vi "Automatic Teller Machine (ATM).vi"() -> ()   [LabVIEW 2020]
doc: "This is my ATM machine"
uses:
  Controls/Ctrl_states.ctl
  Controls/Ctrl_local.ctl
  Controls/Ctrl_UI_Ref.ctl
  <vilib>/Utility/file.llb/Read Delimited Spreadsheet (string).vi
  <vilib>/Utility/file.llb/Write Delimited Spreadsheet (string).vi
panel:
  in  "Enter":bool
  in  "User Input":string
  in  "Right Buttons":T1
  out "Right Menu":T2
  in  "Left Buttons":T1
  out "Left Menu":T2
  in  "Card Simulator":bool
  out "ATM Messages":string
  out "error out":errorcluster caption="sortie d'erreur"
  in  "error in":errorcluster caption="entrée d'erreur"
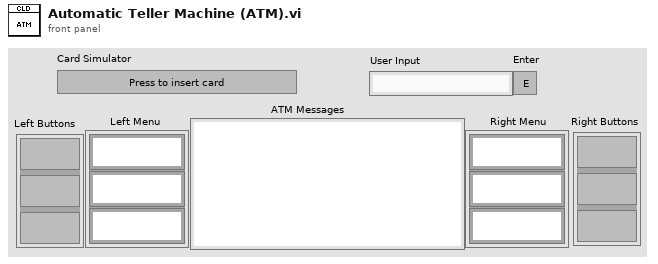
[diagram p1: front panel]
types:
  T1 = cluster{"Func Button":bool, "Func Button 2":bool, "Func Button 3":bool}
  T2 = cluster{"RFS String":string, "RFS String 2":string, "RFS String 3":string}
  T3 = typedef "Ctrl_states.ctl" = enum16{"Account exist", "Account not exist", "Balance Inquiry", "Card inserted", "Display", "Deposit", "Error", "Enter", "Fast Cash", "Read FIle", "Idle", "Init", "Return Card and Terminate", "Save file", "Stop", "Start", "Terminate", "Withdraw"}
  T4 = enum8{"Enabled", "Disabled", "Disabled and Grayed Out"}
  T5 = typedef "Ctrl_local.ctl" = cluster{"State":T3, "Ref":T6, "ATM message":string, "Data":string[][], "User_Input":string, "User_idx":i32, "Terminate ?":bool, "Left Menu":cluster{"RFS String":string, "RFS String 2":string, "RFS String 3":string}, "Right Menu":cluster{"RFS String":string, "RFS String 2":string, "RFS String 3":string}, "Context":T3, "File path":path, "error in":errorcluster}
  T6 = typedef "Ctrl_UI_Ref.ctl" = cluster{"User Input":refnum<vi>, "Enter":refnum<vi>, "Right Buttons":refnum<vi>, "Right Menu":refnum<vi>, "Left Buttons":refnum<vi>, "Left Menu":refnum<vi>, "Card Simulator":refnum<vi>}
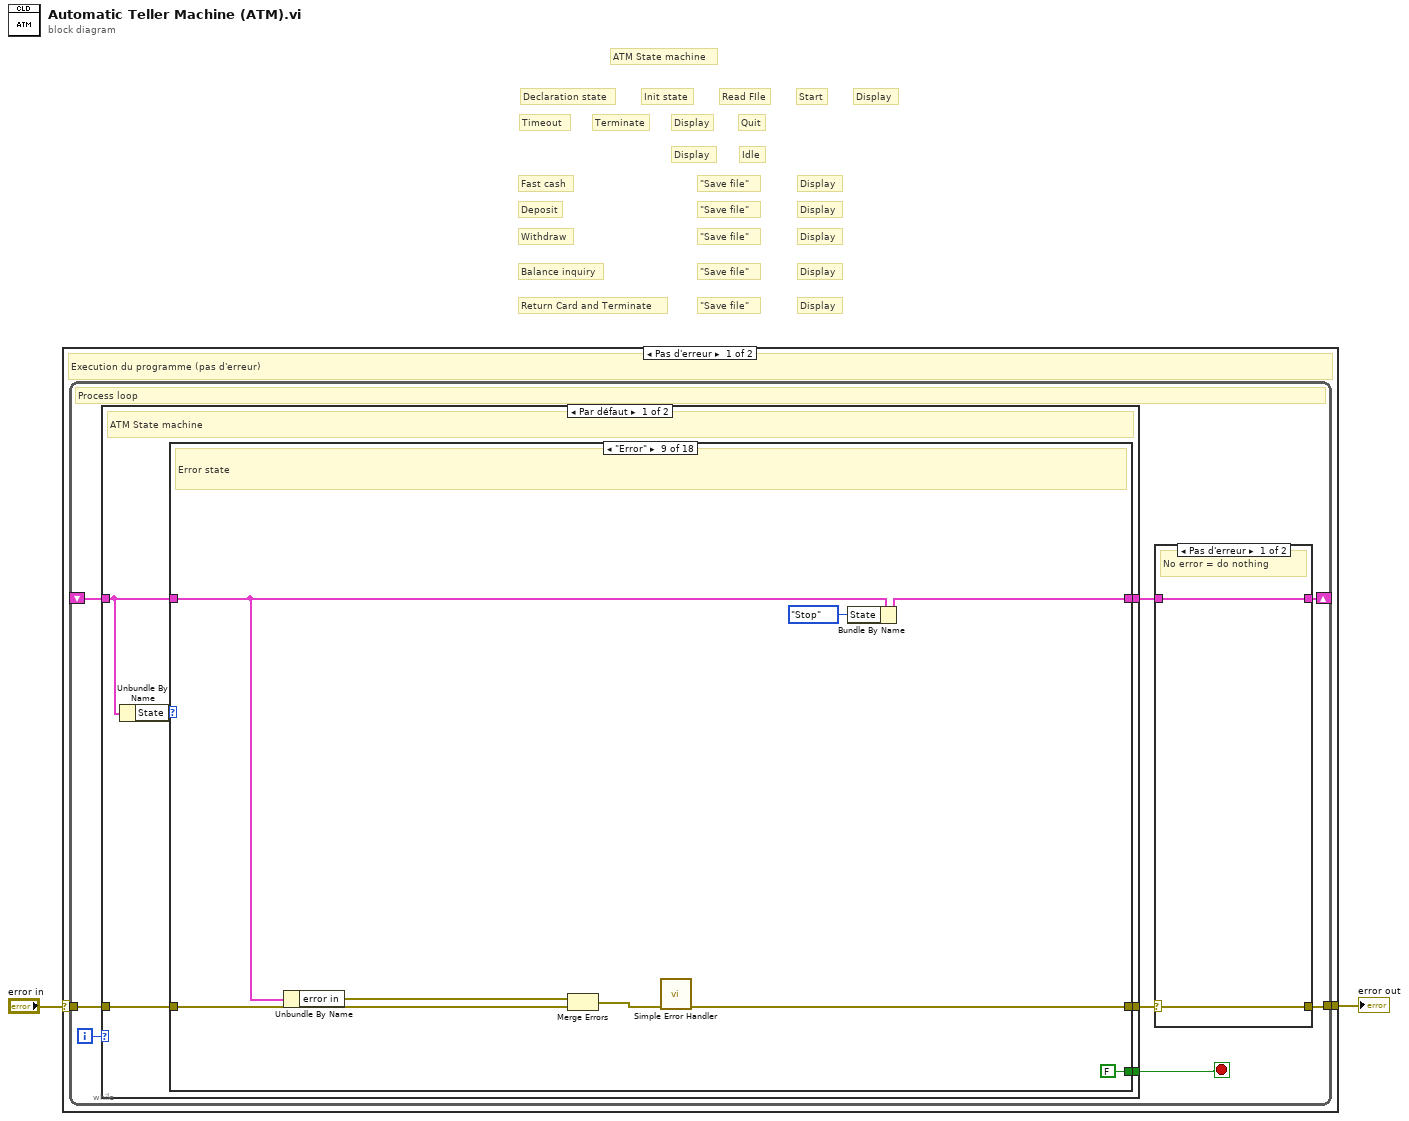
[diagram p0: block diagram]
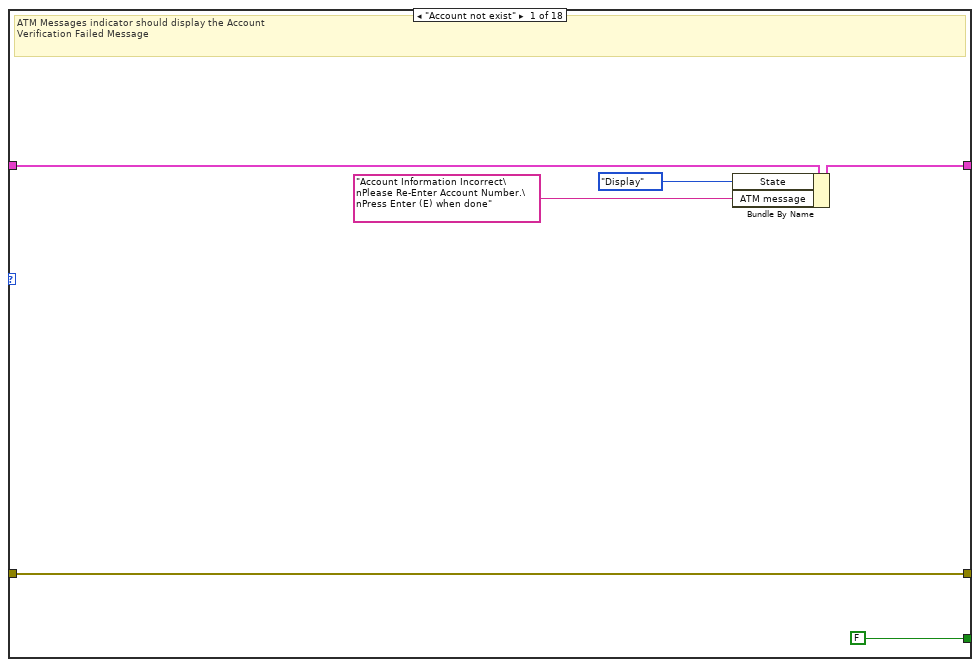
[diagram p2: hidden frame]
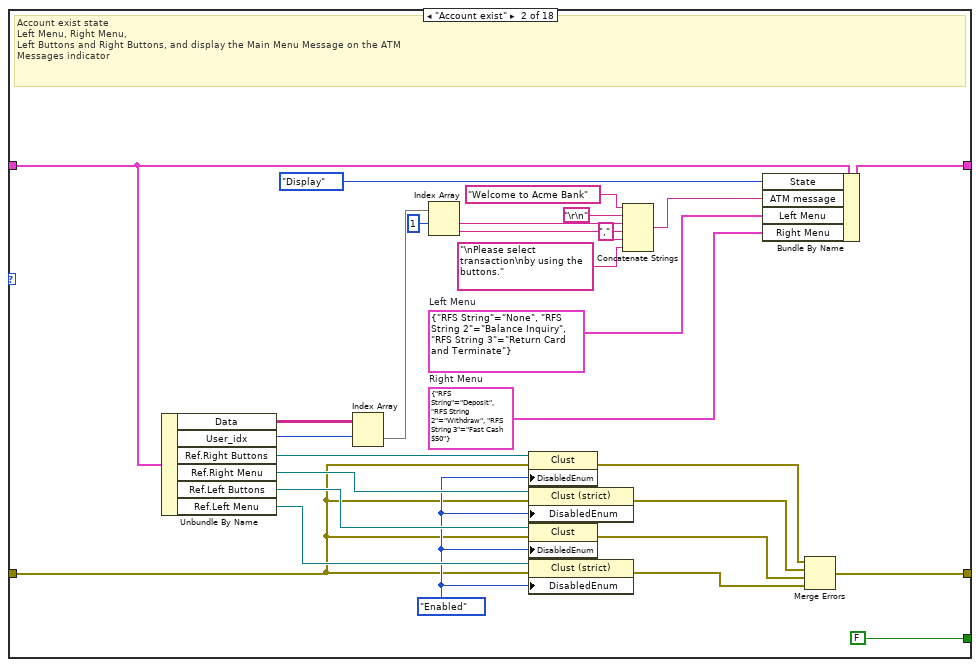
[diagram p3: hidden frame]
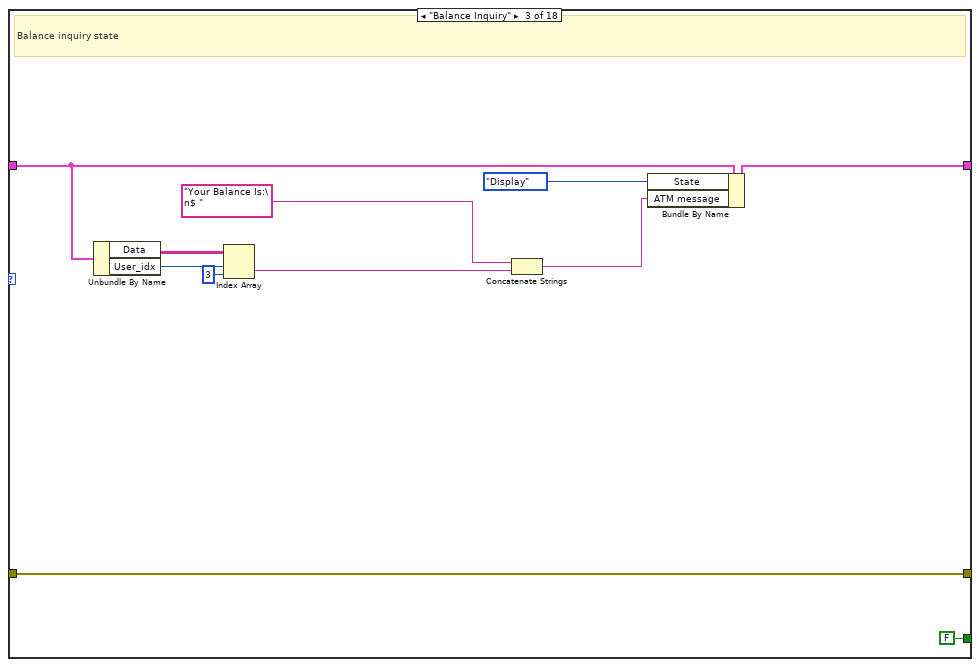
[diagram p4: hidden frame]
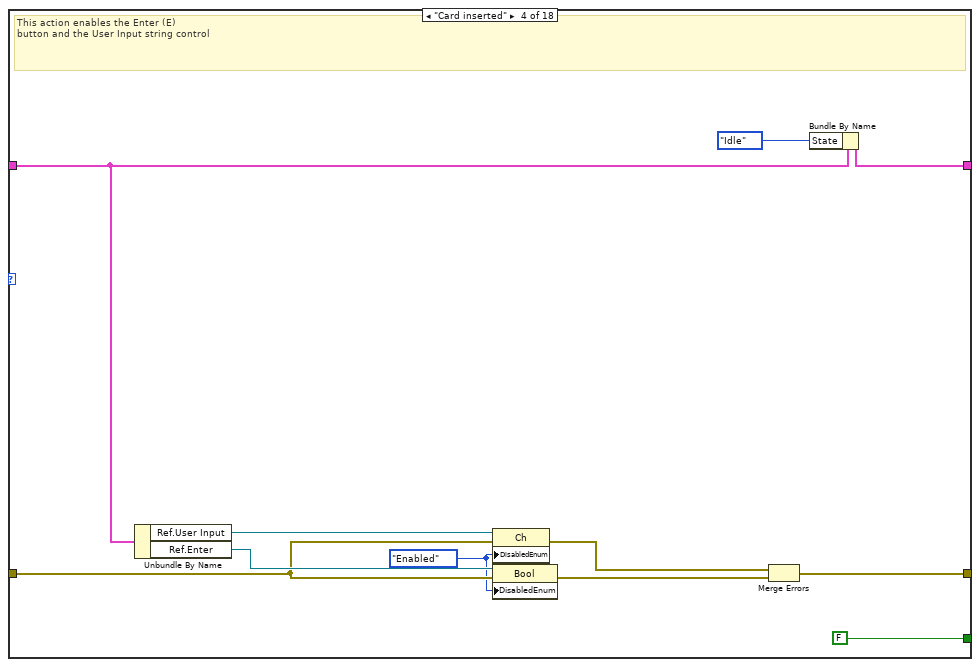
[diagram p5: hidden frame]
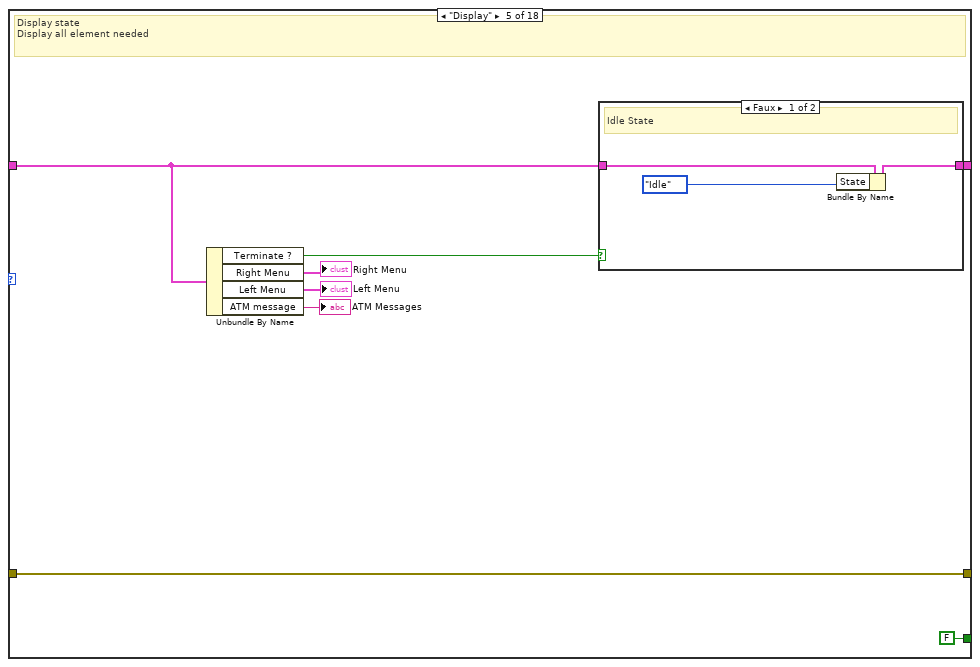
[diagram p6: hidden frame]
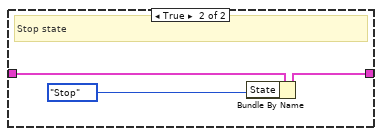
[diagram p7: hidden frame]
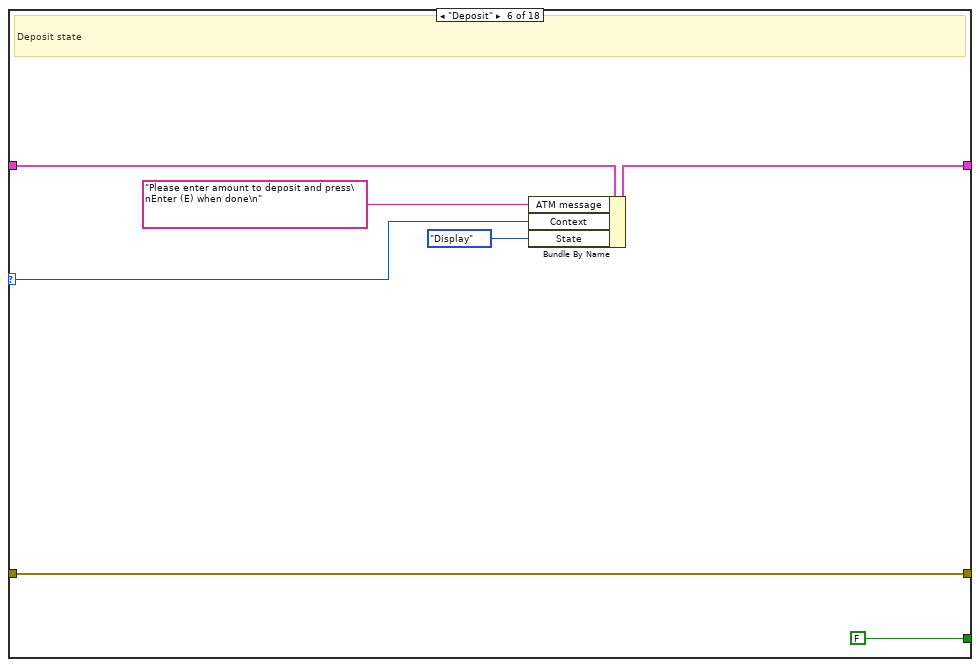
[diagram p8: hidden frame]
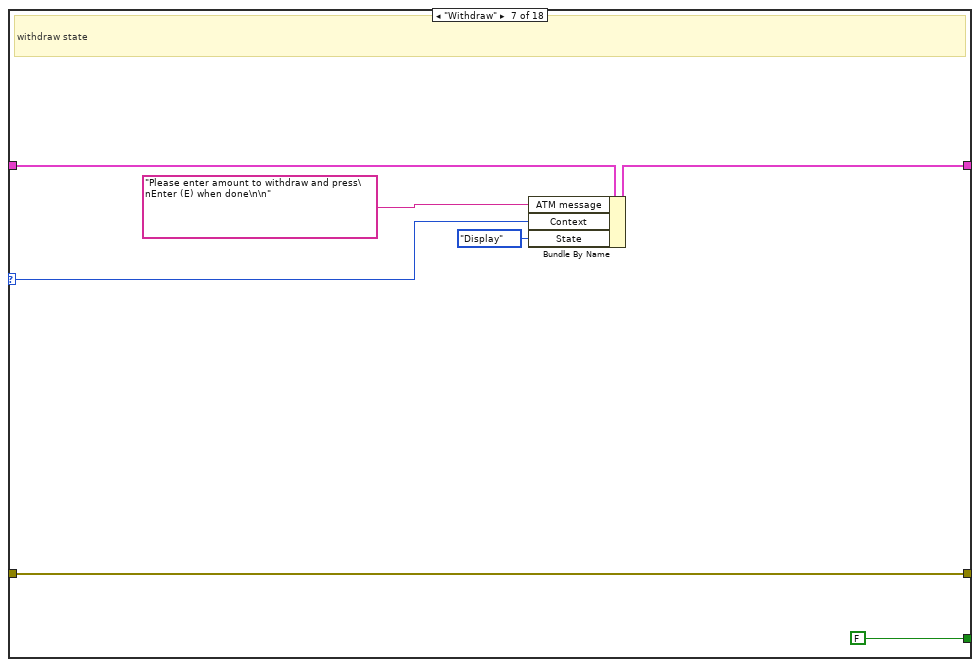
[diagram p9: hidden frame]
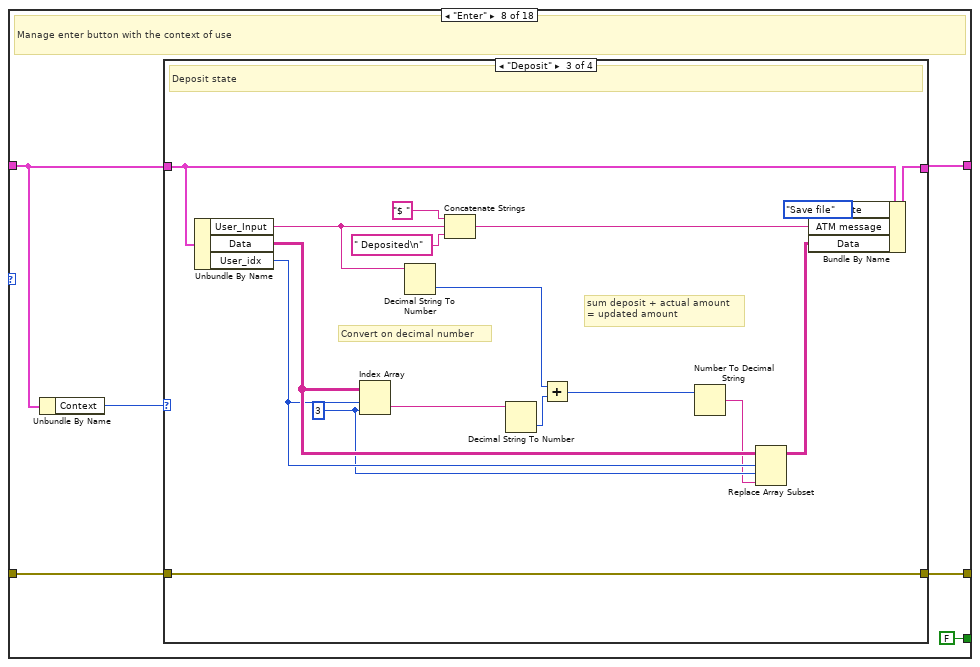
[diagram p10: hidden frame]
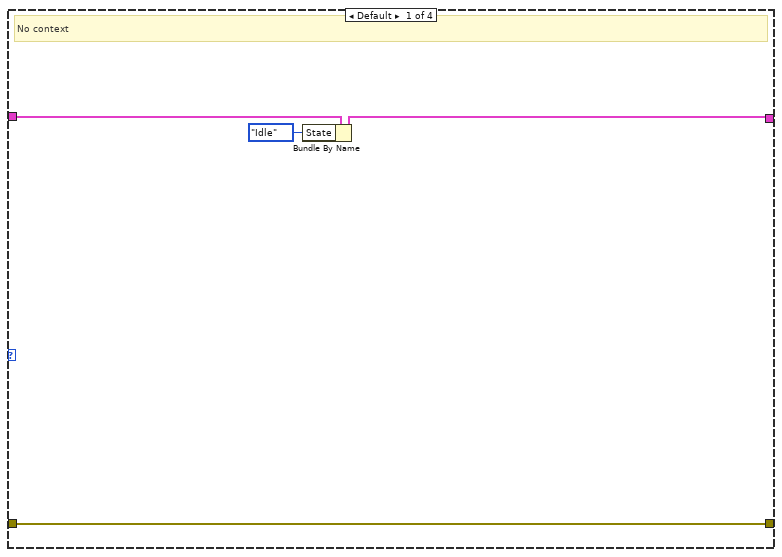
[diagram p11: hidden frame]
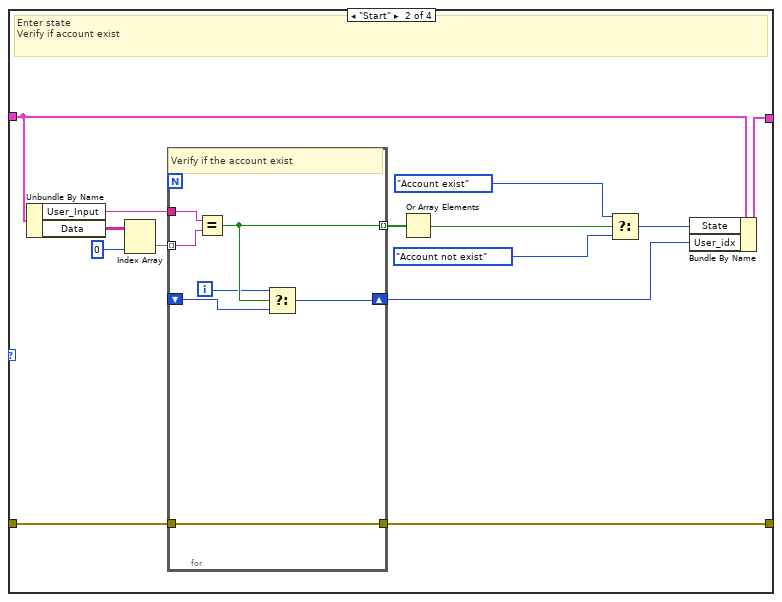
[diagram p12: hidden frame]
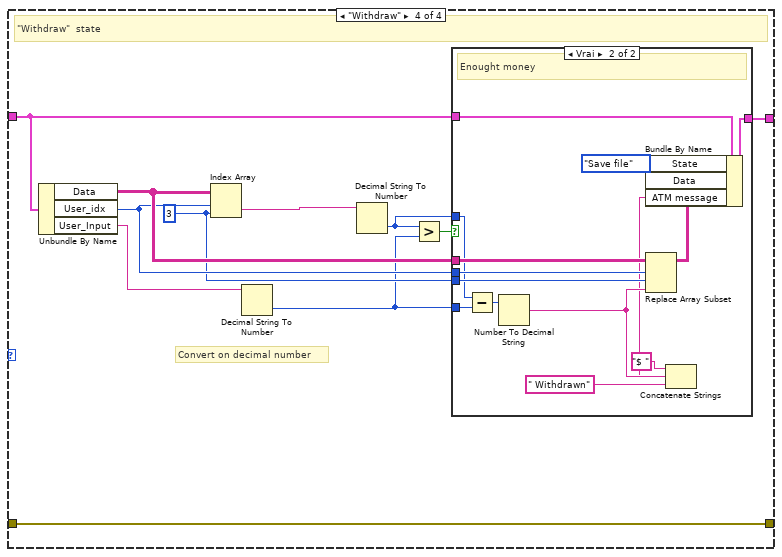
[diagram p13: hidden frame]
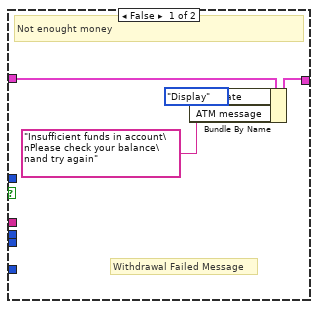
[diagram p14: hidden frame]
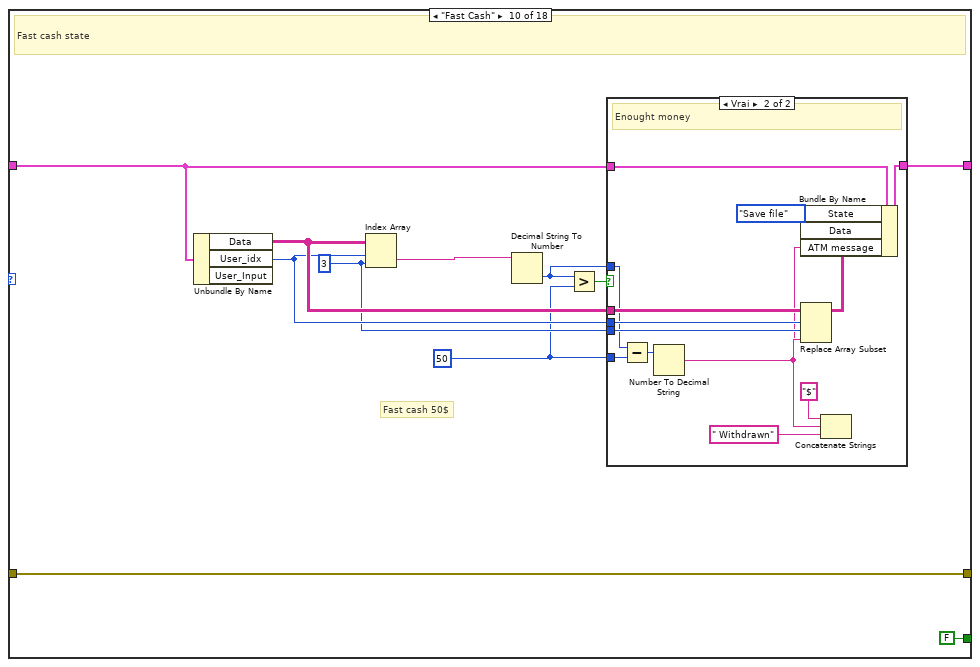
[diagram p15: hidden frame]
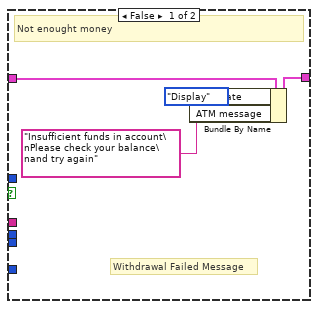
[diagram p16: hidden frame]
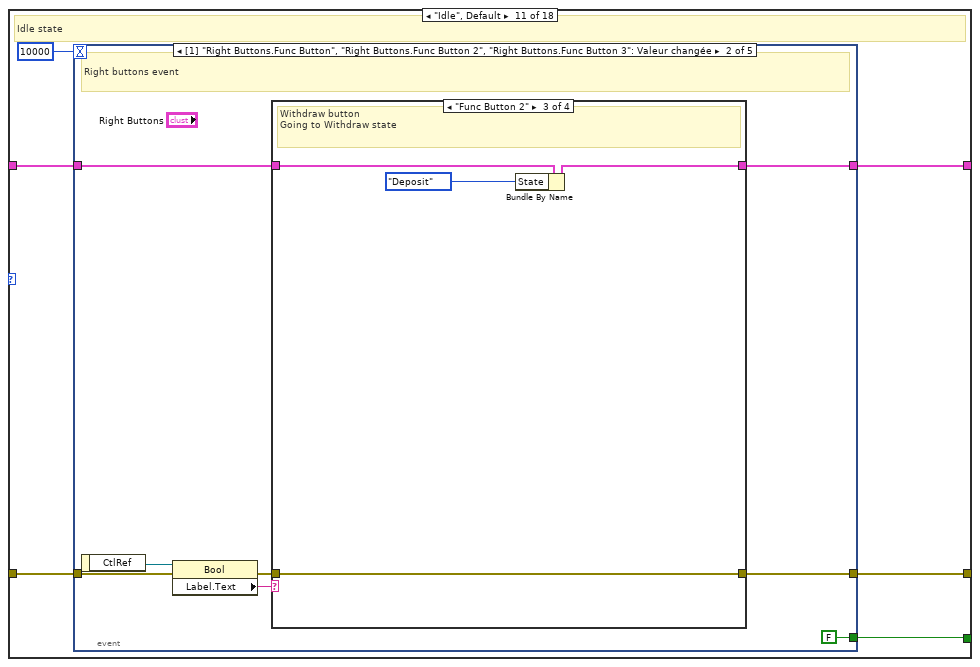
[diagram p17: hidden frame]
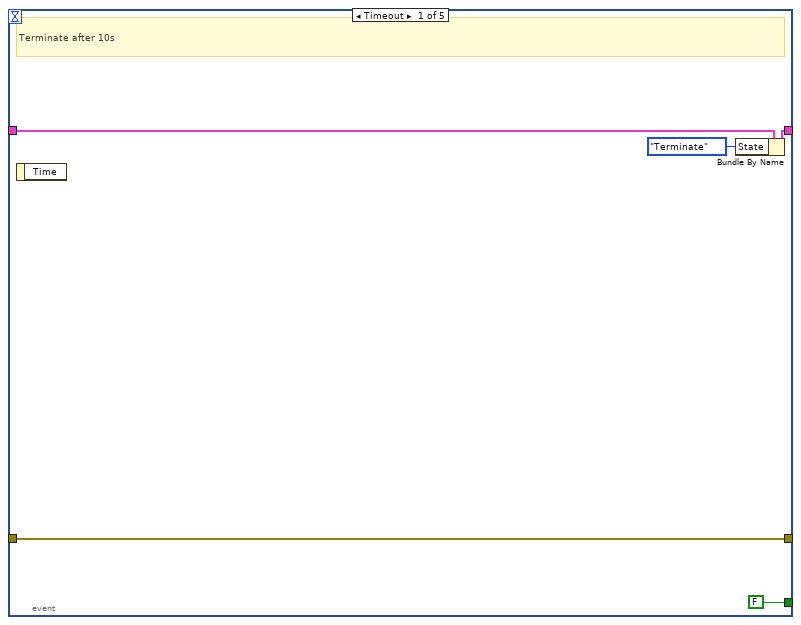
[diagram p18: hidden frame]
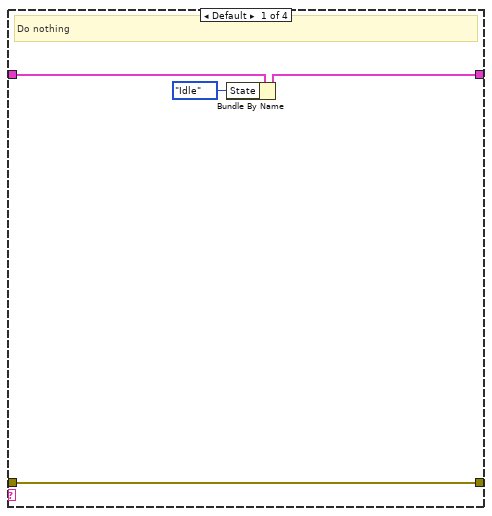
[diagram p19: hidden frame]
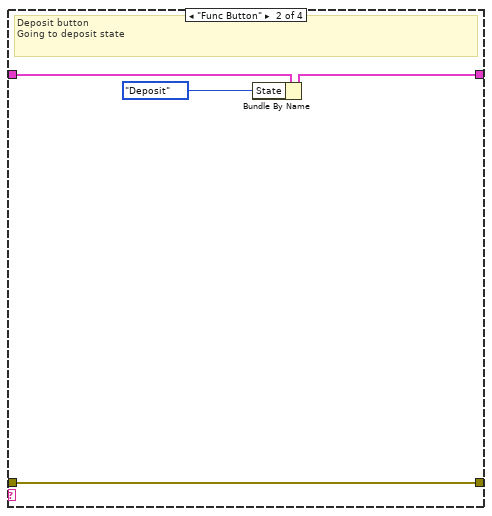
[diagram p20: hidden frame]
diagram:
  # "Display"
  # "\"Save file\""
  # "Display"
  # "\"Save file\""
  # "Display"
  # "\"Save file\""
  # "Display"
  # "\"Save file\""
  # "Display"
  # "\"Save file\""
  # "Read FIle"
  # "Return Card and Terminate"
  # "Balance inquiry"
  # "Withdraw"
  # "Deposit"
  # "Fast cash"
  # "Quit"
  # "Display"
  # "Terminate"
  # "Timeout"
  # "Display"
  # "Idle"
  # "Display"
  # "Start"
  # "Init state"
  # "Declaration state"
  # "ATM State machine"
  n1 = case shown="Pas d'erreur" "error in" {
    selector: "error in" -> [w4 w414]
    tunnel: [w3 w414] -> w1
    frame No Error {
      # "Execution du programme (pas d'erreur)"
      n2 = while {
        tunnel: w4 -> [w12]
        tunnel: [w8] -> w3
        shift-right: [w6] -> _
        shift-left: _ -> [w10]
        i -> [w11]
        stop <- w5 stop-if-true
        # "Process loop"
        n3 = case shown="Par défaut" w11 {
          tunnel: w12 -> [w18 w406]
          tunnel: [w16 w399] -> w9
          tunnel: [w17 FALSE] -> w5
          tunnel: [w15 w403] -> w7
          tunnel: w10 -> [w14 _]
          frame Default {
            # "ATM State machine"
            n4 = Unbundle By Name(w14) -> ("State"=w13:T3)
            n5 = case shown="\"Error\"" w13 {
              selector: w13 -> [_ _ _ _ _ w90 w97 _ _ _ _ _ _ _ _ w355 _ _]
              tunnel: w18 -> [w24 w40 w63 w65 w81 w95 w102 w107 w182 w197 w222 w317 w322 w330 w346 w358 w380 w391]
              tunnel: [FALSE FALSE FALSE ("Release") FALSE FALSE ("Release") FALSE ("Release") FALSE ("Release") FALSE FALSE ("Release") FALSE w221 FALSE FALSE FALSE TRUE FALSE FALSE FALSE] -> w17
              tunnel: [w24 w38 w63 w68 w81 w95 w102 w106 w181 w197 w220 w317 w321 w329 w345 w363 w380 w387] -> w16
              tunnel: w14 -> [w23 w39 w60 w74 w82 w94 w101 w104 w187 w195 w219 w316 w320 w333 w337 w378 w386 w398]
              tunnel: [w22 w52 w62 w67 w80 w93 w100 w105 w186 w196 w218 w315 w327 w336 w337 w362 w384 w396] -> w15
              frame "Account not exist" {
                # "ATM Messages indicator should display the Account\nVerification Failed Message"
                n6 = Bundle By Name(cluster=w23, "State"=Ctrl_states."Display", "ATM message"="Account Information Incorrect\nPlease Re-Enter Account Number.\nPress Enter (E) when done") -> (w22:T5)
              }
              frame "Account exist" {
                w25 = T2 {"RFS String"="Deposit", "RFS String 2"="Withdraw", "RFS String 3"="Fast Cash $50"}  # Right Menu
                w26 = T2 {"RFS String"="None", "RFS String 2"="Balance Inquiry", "RFS String 3"="Return Card and Terminate"}  # Left Menu
                w45 = T4."Enabled" ("Désactivé")
                # "Account exist state\nLeft Menu, Right Menu,\nLeft Buttons and Right Buttons, and display the Main Menu Message on the ATM\nMessages indicator"
                n7 = Unbundle By Name(w39) -> ("Data"=w37:string[][], "User_idx"=w36:i32, "Ref.Right Buttons"=w49:refnum<vi>, "Ref.Right Menu"=w48:refnum<vi>, "Ref.Left Buttons"=w47:refnum<vi>, "Ref.Left Menu"=w46:refnum<vi>)
                n8 = Index Array(array=w37, index (row)=w36) -> (element=w35:string[])  [unwired: 1 in]
                n9 = Index Array(array=w35, index #1=1 ("indice")) -> (element #1=w33:string, element #2=w31:string)  [unwired: 1 in]
                n10 = property class="Clust"(reference=w49, error in=w40, "DisabledEnum"=w45) -> (error out=w44:errorcluster)  [unwired: 1 out]
                n11 = property class="Clust (strict)"(reference=w48, error in=w40, "DisabledEnum"=w45) -> (error out=w43:errorcluster)  [unwired: 1 out]
                n12 = property class="Clust"(reference=w47, error in=w40, "DisabledEnum"=w45) -> (error out=w42:errorcluster)  [unwired: 1 out]
                n13 = property class="Clust (strict)"(reference=w46, error in=w40, "DisabledEnum"=w45) -> (error out=w41:errorcluster)  [unwired: 1 out]
                n14 = Concatenate Strings("Welcome to Acme Bank" ("ATM message"), "\r\n", w33, "," ("chaîne"), w31, "\nPlease select transaction\nby using the buttons." ("ATM message")) -> (w29:string)
                n15 = Bundle By Name(cluster=w39, "State"=Ctrl_states."Display", "ATM message"=w29, "Left Menu"=w26, "Right Menu"=w25) -> (w52:T5)
                n16 = Merge Errors(w44, w43, w42, w41) -> (w38:errorcluster)
              }
              frame "Balance Inquiry" {
                # "Balance inquiry state"
                n17 = Unbundle By Name(w60) -> ("Data"=w59:string[][], "User_idx"=w58:i32)
                n18 = Index Array(array=w59, index (row)=w58, index (col)=3 ("indice désactivé (col)")) -> (element=w55:string)
                n19 = Concatenate Strings("Your Balance Is:\n$ ", w55) -> (w54:string)
                n20 = Bundle By Name(cluster=w60, "State"=Ctrl_states."Display", "ATM message"=w54) -> (w62:T5)
              }
              frame "Card inserted" {
                w64 = T4."Enabled" ("Désactivé")
                # "This action enables the Enter (E)\nbutton and the User Input string control"
                n21 = Unbundle By Name(w74) -> ("Ref.User Input"=w73:refnum<vi>, "Ref.Enter"=w71:refnum<vi>)
                n22 = property class="Ch"(reference=w73, error in=w65, "DisabledEnum"=w64) -> (error out=w70:errorcluster)  [unwired: 1 out]
                n23 = property class="Bool"(reference=w71, error in=w65, "DisabledEnum"=w64) -> (error out=w69:errorcluster)  [unwired: 1 out]
                n24 = Merge Errors(w70, w69) -> (w68:errorcluster)
                n25 = Bundle By Name(cluster=w74, "State"=Ctrl_states."Idle") -> (w67:T5)
              }
              frame "Display" {
                # "Display state\nDisplay all element needed"
                n26 = Unbundle By Name(w82) -> ("Terminate ?"=w75:bool, "Right Menu"=→"Right Menu":T2, "Left Menu"=→"Left Menu":T2, "ATM message"=→"ATM Messages":string)
                n27 = case shown="Faux" w75 {
                  tunnel: w82 -> [w85 w88]
                  tunnel: [w84 w87] -> w80
                  frame False {
                    # "Idle State"
                    n28 = Bundle By Name(cluster=w85, "State"=Ctrl_states."Idle") -> (w84:T5)
                  }
                  frame True {
                    # "Stop state"
                    n29 = Bundle By Name(cluster=w88, "State"=Ctrl_states."Stop") -> (w87:T5)
                  }
                }
              }
              frame "Deposit" {
                # "Deposit state"
                n30 = Bundle By Name(cluster=w94, "ATM message"="Please enter amount to deposit and press\nEnter (E) when done\n", "Context"=w90, "State"=Ctrl_states."Display") -> (w93:T5)
              }
              frame "Withdraw" {
                # "withdraw state"
                n31 = Bundle By Name(cluster=w101, "ATM message"="Please enter amount to withdraw and press\nEnter (E) when done\n\n", "Context"=w97, "State"=Ctrl_states."Display") -> (w100:T5)
              }
              frame "Enter" {
                # "Manage enter button with the context of use"
                n32 = Unbundle By Name(w104) -> ("Context"=w103:T3)
                n33 = case shown="\"Deposit\"" w103 {
                  tunnel: w107 -> [w111 w123 w150 w161]
                  tunnel: [w111 w122 w150 w161] -> w106
                  tunnel: [w110 w119 w149 w154] -> w105
                  tunnel: w104 -> [w112 w113 w147 w155]
                  frame Default {
                    # "No context"
                    n34 = Bundle By Name(cluster=w112, "State"=Ctrl_states."Idle") -> (w110:T5)
                  }
                  frame "Start" {
                    # "Enter state\nVerify if account exist"
                    n35 = Unbundle By Name(w113) -> ("User_Input"=w121:string, "Data"=w126:string[][])
                    n36 = Index Array(array=w126, index (col)=0 ("indice désactivé (col)")) -> (element=w124:string[])  [unwired: 1 in]
                    n37 = for {
                      tunnel: w124 -> [w131] mode=indexing
                      tunnel: w123 -> [w133]
                      tunnel: [w133] -> w122
                      tunnel: w121 -> [w132]
                      tunnel: [w129] -> w120 mode=indexing
                      shift-right: [w130] -> w114
                      shift-left: _ -> [w127]
                      i -> [w128]
                      # "Verify if the account exist"
                      n38 = Equal?(x=w132, y=w131) -> (x = y?=w129:bool)
                      n39 = Select(t=w128, s=w129, f=w127) -> (s? t:f=w130:i32)
                    }
                    n40 = Or Array Elements(Boolean array=w120) -> (logical OR=w118:bool)
                    n41 = Select(t=Ctrl_states."Account exist" ("State"), s=w118, f=Ctrl_states."Account not exist" ("State")) -> (s? t:f=w115:T3)
                    n42 = Bundle By Name(cluster=w113, "State"=w115, "User_idx"=w114) -> (w119:T5)
                  }
                  frame "Deposit" {
                    w137 = 3 ("indice désactivé (col)")
                    # "sum deposit + actual amount\n= updated amount"
                    # "Convert on decimal number"
                    # "Deposit state"
                    n43 = Unbundle By Name(w147) -> ("User_Input"=w143:string, "Data"=w139:string[][], "User_idx"=w138:i32)
                    n44 = Index Array(array=w139, index (row)=w138, index (col)=w137) -> (element=w142:string)
                    n45 = Decimal String To Number(string=w143) -> (number=w140:i32)  [unwired: 2 in, 1 out]
                    n46 = Concatenate Strings("$ ", w143, " Deposited\n") -> (w144:string)
                    n47 = Decimal String To Number(string=w142) -> (number=w141:i32)  [unwired: 2 in, 1 out]
                    n48 = Add(x=w140, y=w141) -> (x+y=w136:i32)
                    n49 = Number To Decimal String(number=w136) -> (decimal integer string=w135:string)  [unwired: 1 in]
                    n50 = Replace Array Subset(array=w139, new element=w135, index (row)=w138, index (col)=w137) -> (w134:string[][])
                    n51 = Bundle By Name(cluster=w147, "State"=Ctrl_states."Save file", "ATM message"=w144, "Data"=w134) -> (w149:T5)
                  }
                  frame "Withdraw" {
                    w157 = 3 ("indice désactivé (col)")
                    # "Convert on decimal number"
                    # "\"Withdraw\"  state"
                    n52 = Unbundle By Name(w155) -> ("Data"=w159:string[][], "User_idx"=w158:i32, "User_Input"=w156:string)
                    n53 = Index Array(array=w159, index (row)=w158, index (col)=w157) -> (element=w160:string)
                    n54 = Decimal String To Number(string=w156) -> (number=w151:i32)  [unwired: 2 in, 1 out]
                    n55 = Decimal String To Number(string=w160) -> (number=w152:i32)  [unwired: 2 in, 1 out]
                    n56 = Greater?(x=w152, y=w151) -> (0:w153:bool)
                    n57 = case shown="Vrai" w153 {
                      tunnel: w159 -> [_ w178]
                      tunnel: w158 -> [_ w177]
                      tunnel: w157 -> [_ w176]
                      tunnel: w155 -> [w165 w174]
                      tunnel: [w164 w173] -> w154
                      tunnel: w152 -> [_ w172]
                      tunnel: w151 -> [_ w171]
                      frame False {
                        # "Withdrawal Failed Message"
                        # "Not enought money"
                        n58 = Bundle By Name(cluster=w165, "State"=Ctrl_states."Display", "ATM message"="Insufficient funds in account\nPlease check your balance\nand try again") -> (w164:T5)
                      }
                      frame True {
                        # "Enought money"
                        n59 = Subtract(x=w172, y=w171) -> (x-y=w170:i32)
                        n60 = Number To Decimal String(number=w170) -> (decimal integer string=w168:string)  [unwired: 1 in]
                        n61 = Replace Array Subset(array=w178, new element=w168, index (row)=w177, index (col)=w176) -> (w175:string[][])
                        n62 = Concatenate Strings("$ ", w168, " Withdrawn" ("chaîne")) -> (w167:string)
                        n63 = Bundle By Name(cluster=w174, "State"=Ctrl_states."Save file", "Data"=w175, "ATM message"=w167) -> (w173:T5)
                      }
                    }
                  }
                }
              }
              frame "Error" {
                # "Error state"
                n64 = Unbundle By Name(w187) -> ("error in"=w184:errorcluster)
                n65 = Merge Errors(w184, w182) -> (w183:errorcluster)
                n66 = call <vilib>:"Simple Error Handler.vi"("error in (no error)"=w183) -> ("error out"=w181:errorcluster)  [unwired: 4 in, 4 out]
                n67 = Bundle By Name(cluster=w187, "State"=Ctrl_states."Stop") -> (w186:T5)
              }
              frame "Fast Cash" {
                w188 = 50 ("y")
                w191 = 3 ("indice désactivé (col)")
                # "Fast cash 50$"
                # "Fast cash state"
                n68 = Unbundle By Name(w195) -> ("Data"=w193:string[][], "User_idx"=w192:i32)  [unwired: 1 out]
                n69 = Index Array(array=w193, index (row)=w192, index (col)=w191) -> (element=w194:string)
                n70 = Decimal String To Number(string=w194) -> (number=w189:i32)  [unwired: 2 in, 1 out]
                n71 = Greater?(x=w189, y=w188) -> (0:w190:bool)
                n72 = case shown="Vrai" w190 {
                  tunnel: w193 -> [_ w215]
                  tunnel: w192 -> [_ w214]
                  tunnel: w191 -> [_ w213]
                  tunnel: w195 -> [w202 w211]
                  tunnel: [w201 w210] -> w196
                  tunnel: w189 -> [_ w209]
                  tunnel: w188 -> [_ w208]
                  frame False {
                    # "Withdrawal Failed Message"
                    # "Not enought money"
                    n73 = Bundle By Name(cluster=w202, "State"=Ctrl_states."Display", "ATM message"="Insufficient funds in account\nPlease check your balance\nand try again") -> (w201:T5)
                  }
                  frame True {
                    # "Enought money"
                    n74 = Subtract(x=w209, y=w208) -> (x-y=w207:i32)
                    n75 = Number To Decimal String(number=w207) -> (decimal integer string=w205:string)  [unwired: 1 in]
                    n76 = Replace Array Subset(array=w215, new element=w205, index (row)=w214, index (col)=w213) -> (w212:string[][])
                    n77 = Concatenate Strings("$", w205, " Withdrawn") -> (w204:string)
                    n78 = Bundle By Name(cluster=w211, "State"=Ctrl_states."Save file", "Data"=w212, "ATM message"=w204) -> (w210:T5)
                  }
                }
              }
              frame "Idle", Default {
                # "Idle state"
                n79 = event shown="[1] \"Right Buttons.Func Button\", \"Right Buttons.Func Button 2\", \"Right Buttons.Func Button 3\": Valeur changée" {
                  selector: _ -> [_ _ _ _ _]
                  dyn-events: _ -> [_ _ _ _ _]
                  timeout: 10000 -> [_ _ _ _ _]
                  tunnel: w222 -> [w226 w234 w258 w281 w287]
                  tunnel: [FALSE FALSE FALSE FALSE FALSE] -> w221
                  tunnel: [w226 w228 w252 w281 w282] -> w220
                  tunnel: w219 -> [w225 w231 w255 w280 w286]
                  tunnel: [w224 w230 w254 w279 w285] -> w218
                  event Timeout {
                    # "Terminate after 10s"
                    n80 = event-data() -> ()  [unwired: 1 in, 1 out]
                    n81 = Bundle By Name(cluster=w225, "State"=Ctrl_states."Terminate") -> (w224:T5)
                  }
                  event "Right Buttons.Func Button", "Right Buttons.Func Button 2", "Right Buttons.Func Button 3": Value Change {
                    # "Right buttons event"
                    n82 = event-data() -> ("CtlRef"=w235:refnum<vi>)  [unwired: 1 in]
                    n83 = property class="Bool"(reference=w235, error in=w234) -> (error out=w229:errorcluster, "Label.Text"=w232:string)  [unwired: 1 out]
                    n84 = case shown="\"Func Button 2\"" w232 {
                      tunnel: w231 -> [w239 w243 w247 w251]
                      tunnel: [w238 w242 w246 w250] -> w230
                      tunnel: w229 -> [w236 w240 w244 w248]
                      tunnel: [w236 w240 w244 w248] -> w228
                      frame Default {
                        # "Do nothing"
                        n85 = Bundle By Name(cluster=w239, "State"=Ctrl_states."Idle") -> (w238:T5)
                      }
                      frame "Func Button" {
                        # "Deposit button\nGoing to deposit state"
                        n86 = Bundle By Name(cluster=w243, "State"=Ctrl_states."Deposit") -> (w242:T5)
                      }
                      frame "Func Button 2" {
                        # "Withdraw button\nGoing to Withdraw state"
                        n87 = Bundle By Name(cluster=w247, "State"=Ctrl_states."Deposit") -> (w246:T5)
                      }
                      frame "Func Button 3" {
                        # "Fast cash button\nGoing to Fast cash state"
                        n88 = Bundle By Name(cluster=w251, "State"=Ctrl_states."Fast Cash") -> (w250:T5)
                      }
                    }
                  }
                  event "Left Buttons.Func Button", "Left Buttons.Func Button 2", "Left Buttons.Func Button 3": Value Change {
                    # "Left buttons event"
                    n89 = event-data() -> ("CtlRef"=w259:refnum<vi>)  [unwired: 1 in]
                    n90 = property class="Bool"(reference=w259, error in=w258) -> (error out=w253:errorcluster, "Label.Text"=w256:string)  [unwired: 1 out]
                    n91 = case shown="\"Func Button 3\"" w256 {
                      tunnel: w255 -> [w263 w267 w271 w275]
                      tunnel: [w262 w266 w270 w274] -> w254
                      tunnel: w253 -> [w260 w264 w268 w272]
                      tunnel: [w260 w264 w268 w272] -> w252
                      frame Default {
                        # "Do nothing"
                        n92 = Bundle By Name(cluster=w263, "State"=Ctrl_states."Idle") -> (w262:T5)
                      }
                      frame "Func Button" {
                        # "none  button\nDo nothing"
                        n93 = Bundle By Name(cluster=w267, "State"=Ctrl_states."Idle") -> (w266:T5)
                      }
                      frame "Func Button 2" {
                        # "Balance inquiry button\nGoing to Balance inquiry state"
                        n94 = Bundle By Name(cluster=w271, "State"=Ctrl_states."Balance Inquiry") -> (w270:T5)
                      }
                      frame "Func Button 3" {
                        # "Return Card and Terminate  button\nGoing to Return Card and Terminate state"
                        n95 = Bundle By Name(cluster=w275, "State"=Ctrl_states."Return Card and Terminate") -> (w274:T5)
                      }
                    }
                  }
                  event "Enter": Value Change {
                    # "Enter state"
                    n96 = event-data() -> ()  [unwired: 1 in, 1 out]
                    n97 = Bundle By Name(cluster=w280, "State"=Ctrl_states."Enter", "User_Input"="User Input") -> (w279:T5)
                  }
                  event "Card Simulator": Value Change {
                    # "Card simulator event"
                    n98 = event-data() -> ("CtlRef"=w288:refnum<vi>)  [unwired: 1 in]
                    n99 = property class="Bool (strict)"(reference=w288, error in=w287) -> (error out=w284:errorcluster, "BoolText.Text"=w283:string)  [unwired: 1 out]
                    n100 = case shown="\"Card inserted\"" w283 {
                      tunnel: w286 -> [w293 w297 w301]
                      tunnel: [w291 w295 w299] -> w285
                      tunnel: w284 -> [w292 w296 w300]
                      tunnel: [w292 w296 w300] -> w282
                      frame Default {
                        # "Default case"
                        n101 = Bundle By Name(cluster=w293, "State"=Ctrl_states."Idle") -> (w291:T5)
                      }
                      frame "Press to insert card" {
                        # "Press to insert card case"
                        n102 = Bundle By Name(cluster=w297, "State"=Ctrl_states."Idle") -> (w295:T5)
                      }
                      frame "Card inserted" {
                        # "Card inserted case"
                        n103 = Bundle By Name(cluster=w301, "State"=Ctrl_states."Card inserted") -> (w299:T5)
                      }
                    }
                  }
                }
              }
              frame "Init" {
                # "Next state"
                # "Initialisation state\nInit all UI references\nSave the file path in the local"
                n104 = Current VI's Path() -> (path=w305:path)
                n105 = Strip Path(path=w305) -> (stripped path=w304:path)  [unwired: 1 out]
                n106 = Build Path(base path=w304, name or relative path=path "ATM accounts.txt" ("nom ou chemin relatif")) -> (appended path=w302:path)
                n107 = control-ref of="Enter"() -> (w312:refnum<vi>)
                n108 = control-ref of="Card Simulator"() -> (w307:refnum<vi>)
                n109 = control-ref of="User Input"() -> (w313:refnum<vi>)
                n110 = control-ref of="Right Buttons"() -> (w311:refnum<vi>)
                n111 = control-ref of="Right Menu"() -> (w310:refnum<vi>)
                n112 = control-ref of="Left Buttons"() -> (w309:refnum<vi>)
                n113 = control-ref of="Left Menu"() -> (w308:refnum<vi>)
                n114 = Bundle By Name(cluster=w316, "State"=Ctrl_states."Read FIle", "Ref.User Input"=w313, "Ref.Enter"=w312, "Ref.Right Buttons"=w311, "Ref.Right Menu"=w310, "Ref.Left Buttons"=w309, "Ref.Left Menu"=w308, "Ref.Card Simulator"=w307, "Terminate ?"=FALSE ("Release"), "File path"=w302) -> (w315:T5)
              }
              frame "Read FIle" {
                # "Next step"
                # "Read the file and store the data in the local"
                n115 = Unbundle By Name(w320) -> ("File path"=w319:path)
                n116 = call-poly <vilib>:"Read Delimited Spreadsheet.vi"("file path (dialog if empty)"=w319, "error in (no error)"=w322, "delimiter (\\t)"="," ("delimiter (\\t)")) -> ("all rows"=w323:string[][], "error out"=w321:errorcluster)  [unwired: 7 in, 4 out]
                n117 = Bundle By Name(cluster=w320, "State"=Ctrl_states."Start", "Data"=w323) -> (w327:T5)
              }
              frame "Save file" {
                # "Save the file with stored data in the local"
                n118 = Unbundle By Name(w333) -> ("File path"=w332:path, "Data"=w331:string[][])
                n119 = call-poly <vilib>:"Write Delimited Spreadsheet.vi"("file path (dialog if empty)"=w332, "2D data"=w331, "error in (no error)"=w330, "delimiter (\\t)"="," ("delimiter (\\t)")) -> ("error out"=w329:errorcluster)  [unwired: 10 in, 1 out]
                n120 = Bundle By Name(cluster=w333, "State"=Ctrl_states."Display") -> (w336:T5)
              }
              frame "Stop" {
                # "Stop state"
                n121 = Unbundle By Name(w337) -> ("Ref.User Input"=w353:refnum<vi>, "Ref.Enter"=w352:refnum<vi>, "Ref.Right Buttons"=w351:refnum<vi>, "Ref.Right Menu"=w350:refnum<vi>, "Ref.Left Buttons"=w349:refnum<vi>, "Ref.Left Menu"=w348:refnum<vi>, "Ref.Card Simulator"=w347:refnum<vi>)
                n122 = Close Reference(reference=w353, error in (no error)=w346) -> (error out=w344:errorcluster)
                n123 = Close Reference(reference=w352, error in (no error)=w346) -> (error out=w343:errorcluster)
                n124 = Close Reference(reference=w351, error in (no error)=w346) -> (error out=w342:errorcluster)
                n125 = Close Reference(reference=w350, error in (no error)=w346) -> (error out=w341:errorcluster)
                n126 = Close Reference(reference=w349, error in (no error)=w346) -> (error out=w340:errorcluster)
                n127 = Close Reference(reference=w348, error in (no error)=w346) -> (error out=w339:errorcluster)
                n128 = Close Reference(reference=w347, error in (no error)=w346) -> (error out=w338:errorcluster)
                n129 = Merge Errors(w344, w343, w342, w341, w340, w339, w338) -> (w345:errorcluster)
              }
              frame "Start" {
                w370 = T4."Disabled and Grayed Out" ("Désactivé")
                # "The User Input, Enter (E), Left\nMenu, Right Menu, Left Buttons, and Right Buttons should be disabled.\nThe Card Simulator button enabled and the ATM Messages indicator should\ndisplay the Welcome Message."
                n130 = Unbundle By Name(w378) -> ("Ref.Card Simulator"=w357:refnum<vi>, "Ref.User Input"=w377:refnum<vi>, "Ref.Enter"=w375:refnum<vi>, "Ref.Right Buttons"=w374:refnum<vi>, "Ref.Right Menu"=w373:refnum<vi>, "Ref.Left Buttons"=w372:refnum<vi>, "Ref.Left Menu"=w371:refnum<vi>)
                n131 = property class="Ch"(reference=w377, error in=w358, "DisabledEnum"=w370) -> (error out=w369:errorcluster)  [unwired: 1 out]
                n132 = property class="Bool"(reference=w375, error in=w358, "DisabledEnum"=w370) -> (error out=w368:errorcluster)  [unwired: 1 out]
                n133 = property class="Clust"(reference=w374, error in=w358, "DisabledEnum"=w370) -> (error out=w367:errorcluster)  [unwired: 1 out]
                n134 = property class="Clust (strict)"(reference=w373, error in=w358, "DisabledEnum"=w370) -> (error out=w366:errorcluster)  [unwired: 1 out]
                n135 = property class="Clust"(reference=w372, error in=w358, "DisabledEnum"=w370) -> (error out=w365:errorcluster)  [unwired: 1 out]
                n136 = property class="Clust (strict)"(reference=w371, error in=w358, "DisabledEnum"=w370) -> (error out=w364:errorcluster)  [unwired: 1 out]
                n137 = property class="Bool (strict)"(reference=w357, error in=w358, "DisabledEnum"=T4."Enabled" ("Désactivé")) -> (error out=w360:errorcluster)  [unwired: 1 out]
                n138 = Merge Errors(w360, w369, w368, w367, w366, w365, w364) -> (w363:errorcluster)
                n139 = Bundle By Name(cluster=w378, "State"=Ctrl_states."Display", "ATM message"="Welcome to Acme Bank.\nPlease insert your card\nand enter your account\nnumber in the User Input.\nPress Enter (E) when done.", "Context"=w355) -> (w362:T5)
              }
              frame "Terminate" {
                w379 = T2 {"RFS String"="", "RFS String 2"="", "RFS String 3"=""} ("Left Menu")
                # "the Card Simulator button should be\nreleased and the user session should be terminated by stopping the application. The ATM\nMessages indicator should display the Session Terminate Message."
                n140 = Bundle By Name(cluster=w386, "State"=Ctrl_states."Display", "ATM message"="Your session has been terminated\ndue to inactivity or menu selection.\nPlease take your card\nGoodbye!\n", "Terminate ?"=TRUE ("Release"), "Left Menu"=w379, "Right Menu"=w379) -> (w384:T5)
              }
              frame "Return Card and Terminate" {
                w390 = T2 {"RFS String"="", "RFS String 2"="", "RFS String 3"=""} ("Left Menu")
                # "Close reference"
                # "The ATM Messages indicator should display the\nSession Terminate Message. The ATM controller should release the Card\nSimulator button to indicate the return of the ATM card, disable the User Input control,\nand terminate the application."
                n141 = control-ref of="Ce VI"() -> (w392:refnum<vi>)
                n142 = invoke class="VI" method="ValsParDéfaut.TtRét"(reference=w392, error in=w391) -> (reference out=w388:refnum<vi>, error out=w389:errorcluster)  [unwired: 1 in, 1 out]
                n143 = Close Reference(reference=w388, error in (no error)=w389) -> (error out=w387:errorcluster)
                n144 = Bundle By Name(cluster=w398, "State"=Ctrl_states."Display", "ATM message"="Your session has been terminated\ndue to inactivity or menu selection.\nPlease take your card\nGoodbye!\n", "Terminate ?"=TRUE ("Release"), "Left Menu"=w390, "Right Menu"=w390) -> (w396:T5)
              }
            }
          }
          frame 0 {
            # "Initialisation du VI\nDeclaration state"
            n145 = control-ref of="Ce VI"() -> (w407:refnum<vi>)
            n146 = invoke class="VI" method="ValsParDéfaut.TtRét"(reference=w407, error in=w406) -> (reference out=w400:refnum<vi>, error out=w401:errorcluster)  [unwired: 1 in, 1 out]
            n147 = Close Reference(reference=w400, error in (no error)=w401) -> (error out=w399:errorcluster)
            n148 = Bundle By Name(cluster=T5 {"State"=enum."Init", "Ref"={"User Input"=refnum, "Enter"=refnum, "Right Buttons"=refnum, "Right Menu"=refnum, "Left Buttons"=refnum, "Left Menu"=refnum, "Card Simulator"=refnum}, "ATM message"="", "Data"=[], "User_Input"="", "User_idx"=0, "Terminate ?"=FALSE, "Left Menu"={"RFS String"="", "RFS String 2"="", "RFS String 3"=""}, "Right Menu"={"RFS String"="", "RFS String 2"="", "RFS String 3"=""}, "Context"=enum."Init", "File path"=path "", "error in"={"status"=FALSE, "code"=0, "source"=""}} ("Local"), "State"=Ctrl_states."Init") -> (w403:T5)
          }
        }
        n149 = case shown="Pas d'erreur" w9 {
          selector: w9 -> [w409 w410]
          tunnel: [w409 w410] -> w8
          tunnel: w7 -> [w408 w413]
          tunnel: [w408 w412] -> w6
          frame No Error {
            # "No error = do nothing"
          }
          frame Error {
            # "Error manage it"
            n150 = Bundle By Name(cluster=w413, "State"=Ctrl_states."Error", "error in"=w410) -> (w412:T5)
          }
        }
      }
    }
    frame Error {
      # "non execution du programme (erreur)"
    }
  }
  "error out" <- w1
